vi "onTestExecution.vi"(6 "timeout (2000 ms)":i32=2000, 7 "Name":string, 8 "error in (no error)":errorcluster, 11 "DMC Test Runner in":refnum<class "DMC Test Runner.lvclass">) -> (0 "error out":errorcluster, 3 "DMC Test Runner out":refnum<class "DMC Test Runner.lvclass">)   [LabVIEW 2023, in "DMC Test Runner.lvclass"]
doc: "Same as standard Caraya Unit Test, but adds in optional verbose CLI logging."
uses:
  DMC Test Runner.lvclass
  <vilib>/addons/_JKI Toolkits/Caraya/classes/Test Runner/Test Runner.lvclass
  <vilib>/addons/_JKI Toolkits/Caraya/classes/Test/Test.lvclass
  <vilib>/addons/_JKI Toolkits/Caraya/classes/Assert/Assert.lvclass
  <vilib>/addons/_JKI Toolkits/Caraya/classes/Assert/Assert Not Error.vi
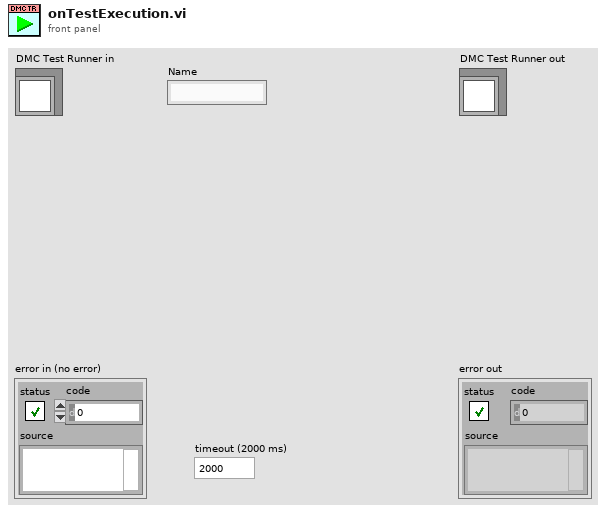
[diagram p1: front panel]
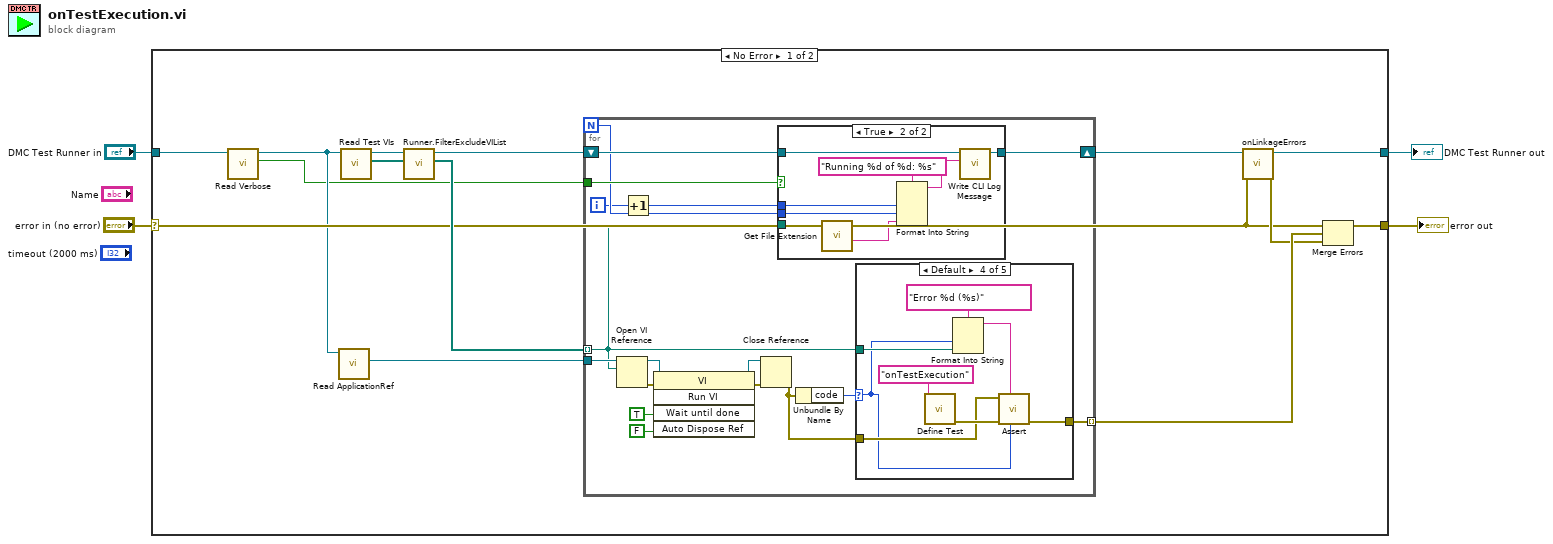
[diagram p0: block diagram]
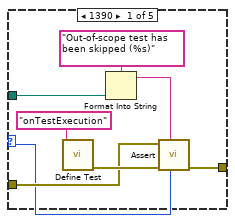
[diagram p3: hidden frame]
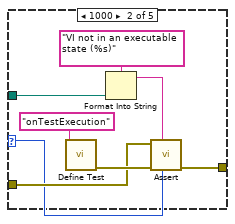
[diagram p4: hidden frame]
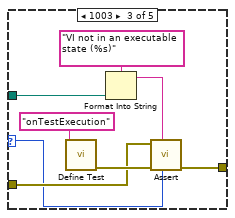
[diagram p5: hidden frame]
diagram:
  n1 = case shown="No Error" "error in (no error)" {
    selector: "error in (no error)" -> [w10 w79]
    tunnel: "DMC Test Runner in" -> [w8 w78]
    tunnel: [w16 w78] -> w1
    tunnel: [w15 w79] -> w2
    frame No Error {
      n2 = call <vilib>:"Read Verbose.vi"("Test Runner in"=w8) -> ("Verbose"=w7:bool, "Test Runner out"=w9:refnum<class "DMC Test Runner.lvclass">)  [unwired: 9 in]
      n3 = call <vilib>:"Read ApplicationRef.vi"("Test Runner in"=w9) -> ("Application"=w17:refnum<vi>)  [unwired: 8 in, 2 out]
      n4 = call <vilib>:"Read Test VIs.vi"("Test Runner in"=w9) -> ("Test VIs"=w13:path[], "Test Runner out"=w11:refnum<class "DMC Test Runner.lvclass">)  [unwired: 8 in, 1 out]
      n5 = call <vilib>:"Runner.FilterExcludeVIList.vi"("Paths"=w13, "Test Runner"=w11) -> ("Filtered Paths"=w12:path[], "Test Runner"=w6:refnum<class "DMC Test Runner.lvclass">)  [unwired: 8 in]
      n6 = for {
        N -> [w23]
        tunnel: w12 -> [w25] mode=indexing
        tunnel: [w35] -> w18 mode=indexing
        tunnel: w17 -> [w34]
        shift-right: [w19] -> w5
        shift-left: w6 -> [w26]
        tunnel: w7 -> [w24]
        i -> [w22]
        n7 = Open VI Reference(application reference (local)=w34, vi path=w25) -> (vi reference=w27:refnum<vi>, error out=w33:errorcluster)  [unwired: 4 in]
        n8 = Increment(x=w22) -> (x+1=w21:i32)
        n9 = invoke on="Invoke Node" class="VI" method="Run VI"(reference=w27, error in=w33, "Wait until done"=TRUE ("Wait Until Done"), "Auto Dispose Ref"=FALSE ("Auto Dispose Reference")) -> (reference out=w29:refnum<vi>, error out=w28:errorcluster)  [unwired: 1 in, 3 out]
        n10 = Close Reference(reference=w29, error in (no error)=w28) -> (error out=w20:errorcluster)
        n11 = case shown="True" w24 {
          tunnel: w26 -> [w36 w41]
          tunnel: [w36 w40] -> w19
          tunnel: w25 -> [_ w43]
          tunnel: w23 -> [_ w38]
          tunnel: w21 -> [_ w37]
          frame False {
          }
          frame True {
            n12 = call <vilib>:"Get File Extension.vi"("file"=w43) -> ("filename without extension"=w42:string)  [unwired: 6 in, 4 out]
            n13 = Format Into String(format string="Running %d of %d: %s", w37, w38, w42) -> (resulting string=w39:string)  [unwired: 2 in, 1 out]
            n14 = call "Write CLI Log Message.vi"("Message"=w39, "DMC Test Runner in"=w41) -> ("DMC Test Runner out"=w40:refnum<class "DMC Test Runner.lvclass">)  [unwired: 8 in, 1 out]
          }
        }
        n15 = Unbundle By Name(w20) -> ("code"=w30:i32)
        n16 = case shown="Default" w30 {
          selector: w30 -> [w45 w53 w61 w69 _]
          tunnel: w20 -> [w46 w54 w62 w70 w77]
          tunnel: [w48 w56 w64 w73 w77] -> w35
          tunnel: w25 -> [w52 w60 w68 w76 _]
          frame 1390 {
            n17 = call <vilib>:"Define Test.vi"("Label (VI Title)"="onTestExecution" ("Label")) -> ("error out"=w49:errorcluster)  [unwired: 9 in, 1 out]
            n18 = Format Into String(format string="Out-of-scope test has been skipped (%s)" ("Label"), w52) -> (resulting string=w47:string)  [unwired: 2 in, 1 out]
            n19 = call-poly <vilib>:"Assert.vi"("error code (1)"=w45, "Label"=w47, "error in (no error)"=w49, "Not Error?"=w46) -> ("error out"=w48:errorcluster)  [unwired: 6 in, 1 out]
          }
          frame 1000 {
            n20 = call <vilib>:"Define Test.vi"("Label (VI Title)"="onTestExecution" ("Label")) -> ("error out"=w57:errorcluster)  [unwired: 9 in, 1 out]
            n21 = Format Into String(format string="VI not in an executable state (%s)" ("Label"), w60) -> (resulting string=w55:string)  [unwired: 2 in, 1 out]
            n22 = call-poly <vilib>:"Assert.vi"("error code (1)"=w53, "Label"=w55, "error in (no error)"=w57, "Not Error?"=w54) -> ("error out"=w56:errorcluster)  [unwired: 6 in, 1 out]
          }
          frame 1003 {
            n23 = call <vilib>:"Define Test.vi"("Label (VI Title)"="onTestExecution" ("Label")) -> ("error out"=w65:errorcluster)  [unwired: 9 in, 1 out]
            n24 = Format Into String(format string="VI not in an executable state (%s)" ("Label"), w68) -> (resulting string=w63:string)  [unwired: 2 in, 1 out]
            n25 = call-poly <vilib>:"Assert.vi"("error code (1)"=w61, "Label"=w63, "error in (no error)"=w65, "Not Error?"=w62) -> ("error out"=w64:errorcluster)  [unwired: 6 in, 1 out]
          }
          frame Default {
            n26 = call <vilib>:"Define Test.vi"("Label (VI Title)"="onTestExecution" ("Label")) -> ("error out"=w71:errorcluster)  [unwired: 9 in, 1 out]
            n27 = Format Into String(format string="Error %d (%s)" ("Label"), w69, w76) -> (resulting string=w72:string)  [unwired: 2 in, 1 out]
            n28 = call-poly <vilib>:"Assert.vi"("error code (1)"=w69, "Label"=w72, "error in (no error)"=w71, "Not Error?"=w70) -> ("error out"=w73:errorcluster)  [unwired: 6 in, 1 out]
          }
          frame 0 {
          }
        }
      }
      n29 = call-dynamic "onLinkageErrors.vi"("error in (no error)"=w10, "Test Runner in"=w5) -> ("error out"=w14:errorcluster, "Test Runner out"=w16:refnum<class "DMC Test Runner.lvclass">)  [unwired: 8 in]
      n30 = Merge Errors(w10, w18, w14) -> (w15:errorcluster)
    }
    frame Error {
    }
  }
  "error out" <- w2
  "DMC Test Runner out" <- w1
